vi "CodeSelet.vi"(11 "parameter name":string="ZP05") -> (3 "readData":string)   [LabVIEW 2013]
uses:
  <vilib>/addons/database/Auxilliary.llb/DB Tools Parameter Dir.ctl
  <vilib>/addons/database/Auxilliary.llb/DB Tools DataTypes.ctl
  <vilib>/addons/database/_DB Variant To Data/Database Variant To Data.xnode
  <vilib>/addons/database/NI_Database_API.lvlib
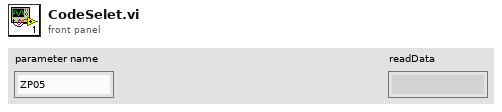
[diagram p1: front panel]
types:
  T1 = typedef "NI_Database_API.lvlib/DB Tools DataTypes.ctl" = enum16{"String", "Long (I32)", "Single (SGL)", "Double (DBL)", "Date/Time", "Binary"}
  T2 = typedef "NI_Database_API.lvlib/DB Tools Parameter Dir.ctl" = enum32{"Input", "Output", "Input/Output", "Return Value"}
  T3 = cluster{"parameter name":string, "type":T1, "direction":T2, "parameter name":string}
  T4 = cluster{"parameter name":string, "type":T1, "direction":T2, "parameter name":string}[]
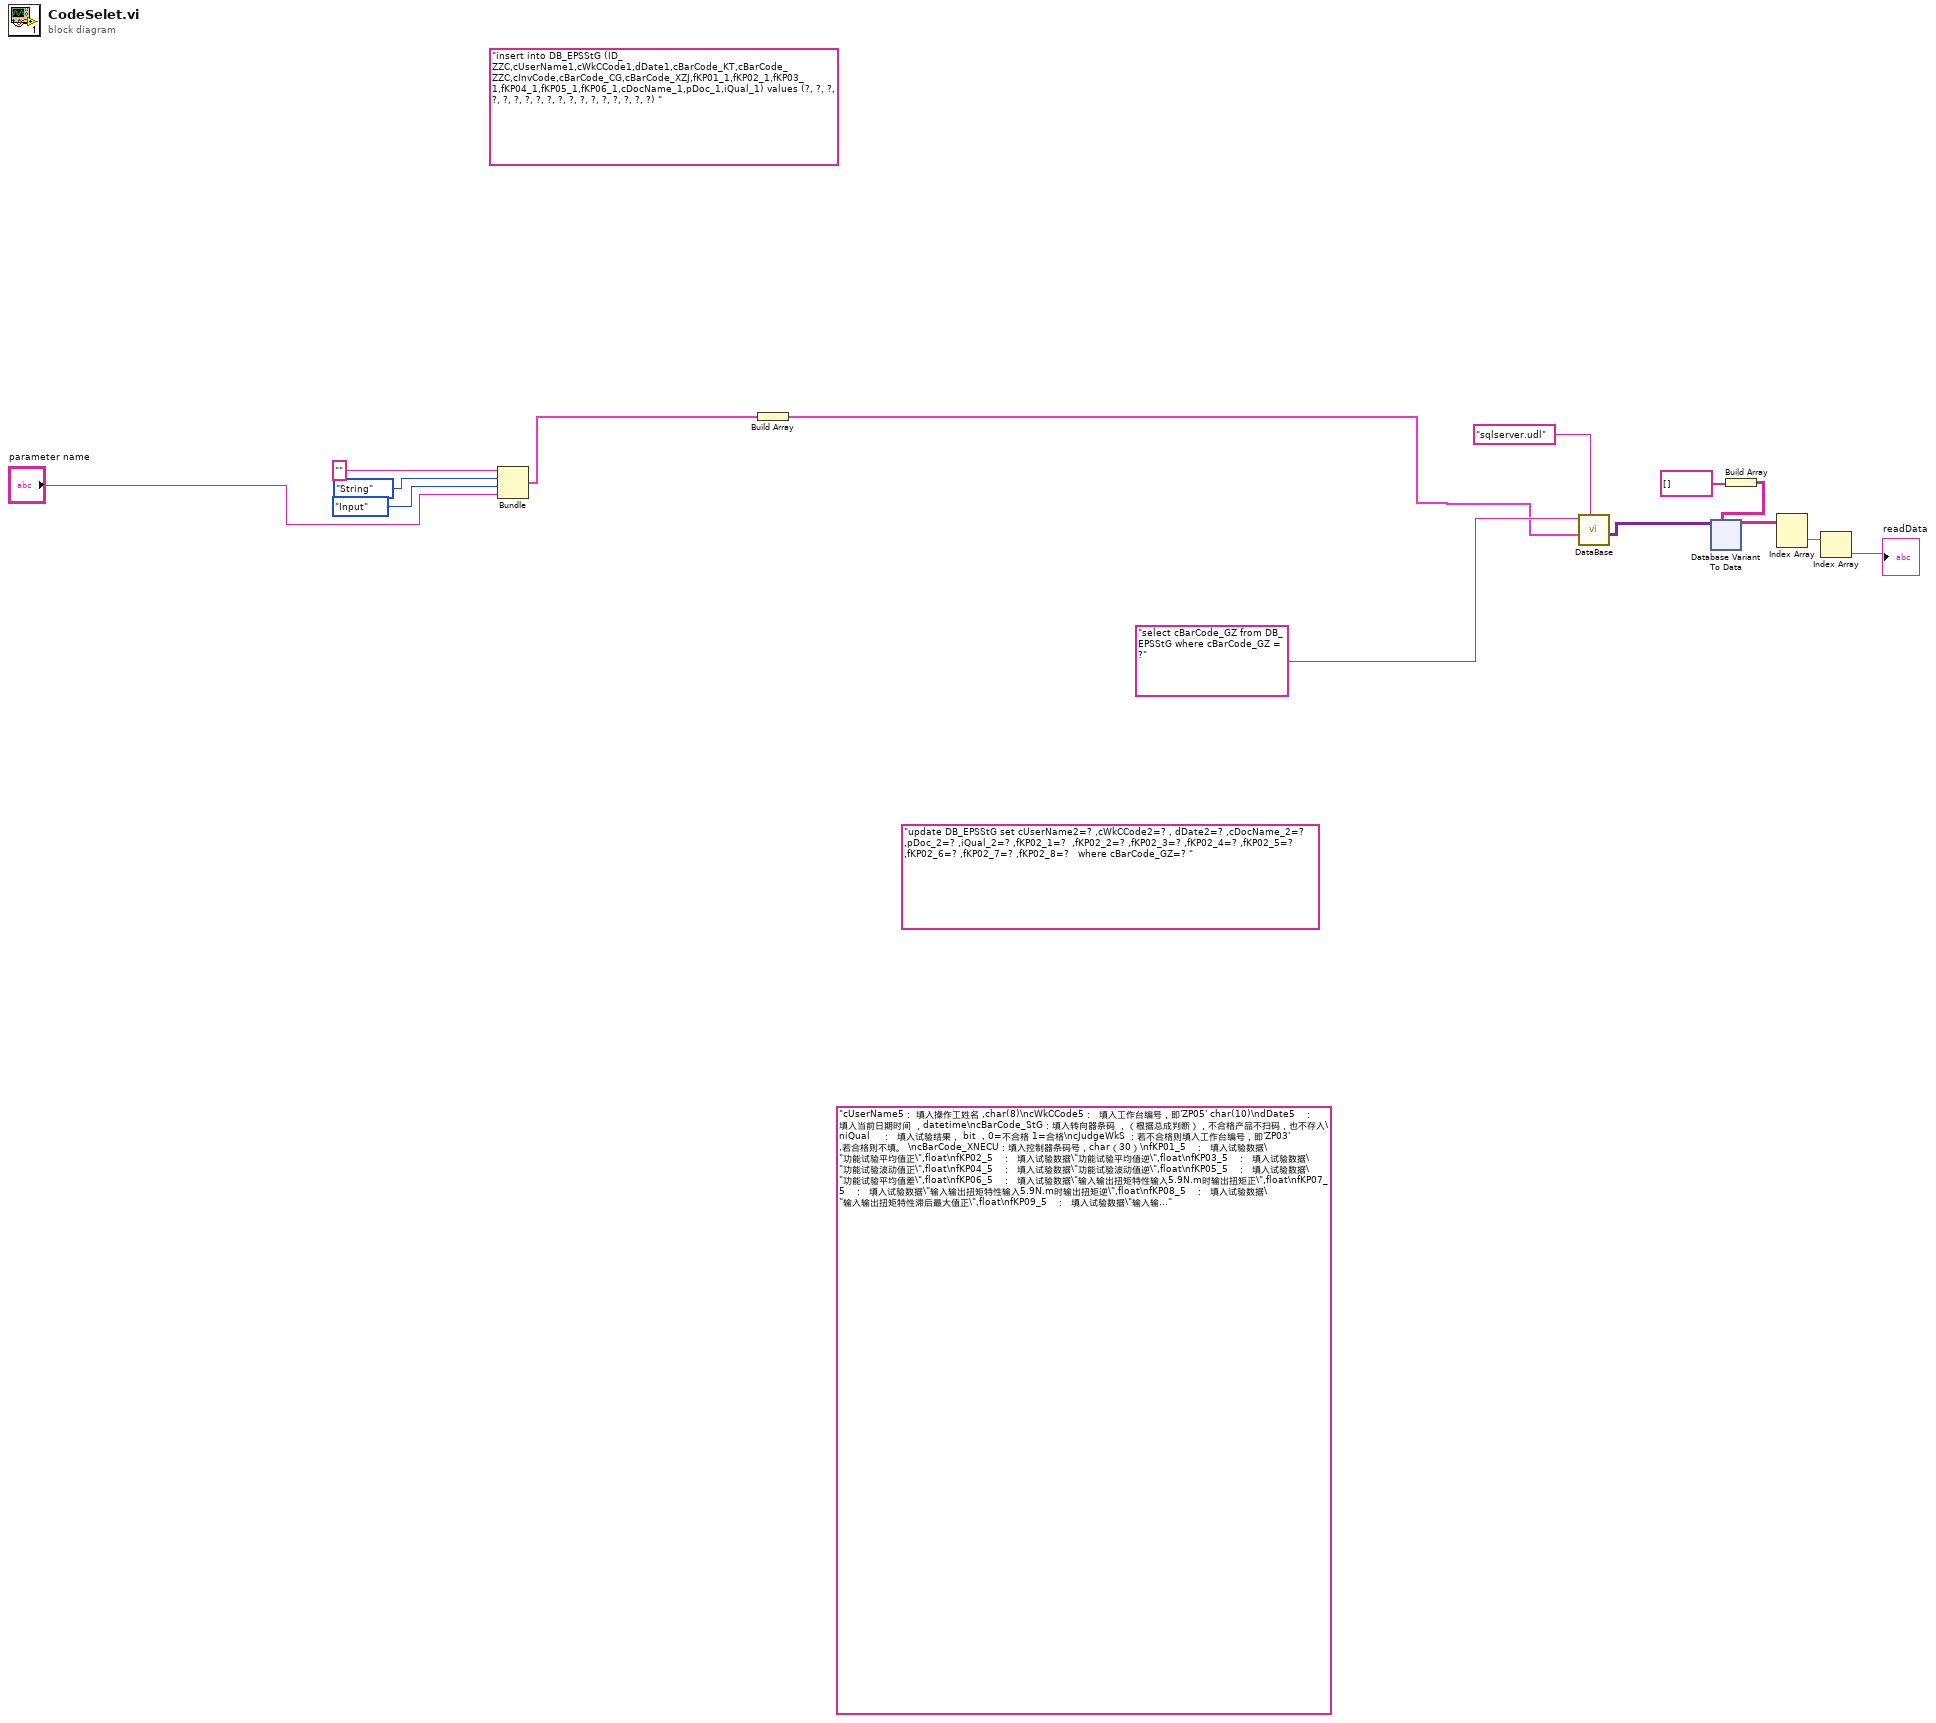
[diagram p0: block diagram]
diagram:
  (unwired) "insert into DB_EPSStG (ID_ZZC,cUserName1,cWkCCode1,dDate1,cBarCode_KT,cBarCode_ZZC,cInvCode,cBarCode_CG,cBarCode_XZJ,fKP01_1,fKP02_1,fKP03_1,fKP04_1,fKP05_1,fKP06_1,cDocName_1,pDoc_1,iQual_1) values (?, ?, ?, ?, ?, ?, ?, ?, ?, ?, ?, ?, ?, ?, ?, ?, ?, ?) " ("SQL query")
  (unwired) "update DB_EPSStG set cUserName2=? ,cWkCCode2=? , dDate2=? ,cDocName_2=? ,pDoc_2=? ,iQual_2=? ,fKP02_1=?  ,fKP02_2=? ,fKP02_3=? ,fKP02_4=? ,fKP02_5=? ,fKP02_6=? ,fKP02_7=? ,fKP02_8=?   where cBarCode_GZ=? " ("SQL query")
  (unwired) "cUserName5： 填入操作工姓名 ,char(8)\ncWkCCode5：  填入工作台编号，即'ZP05' char(10)\ndDate5   ：  填入当前日期时间 ，datetime\ncBarCode_StG：填入转向器条码 ，（根据总成判断），不合格产品不扫码，也不存入\niQual    ：  填入试验结果， bit  , 0=不合格 1=合格\ncJudgeWkS ：若不合格则填入工作台编号，即'ZP03' ,若合格则不填。 \ncBarCode_XNECU：填入控制器条码号，char（30）\nfKP01_5   ：  填入试验数据\"功能试验平均值正\",float\nfKP02_5   ：  填入试验数据\"功能试验平均值逆\",float\nfKP03_5   ：  填入试验数据\"功能试验波动值正\",float\nfKP04_5   ：  填入试验数据\"功能试验波动值逆\",float\nfKP05_5   ：  填入试验数据\"功能试验平均值差\",float\nfKP06_5   ：  填入试验数据\"输入输出扭矩特性输入5.9N.m时输出扭矩正\",float\nfKP07_5   ：  填入试验数据\"输入输出扭矩特性输入5.9N.m时输出扭矩逆\",float\nfKP08_5   ：  填入试验数据\"输入输出扭矩特性滞后最大值正\",float\nfKP09_5   ：  填入试验数据\"输入输出扭矩特性滞后最大值逆\",float\nfKP10_5   ：  填入试验数据\"输入输出扭矩特性对称度\",float\nfKP11_5   ：  填入试验数据\"扭矩传感器特性滞后最大值正\",float\nfKP12_5   ：  填入试验数据\"扭矩传感器特性滞后最大值逆\",float\nfKP13_5   ：  填入试验数据\"扭矩传感器特性对称度\",float\nfKP14_5   ：  填入试验数据\"空载平均值正\",float\nfKP15_5   ：  填入试验数据\"空载平均值逆\",float\nfKP16_5   ：  填入试验数据\"空载平均值差\",float\nfKP17_5   ：  填入试验数据\"空载波动值正\",float\nfKP18_5   ：  填入试验数据\"空载波动值逆\",float\nfKP19_5   ：  填入试验数据\"空载最大值正\",float\nfKP20_5   ：  填入试验数据\"空载最大值逆\",float\n\ncDocName_5：  填入试验报告文件名称，char（40），根据实际文件名，可与本机存储的文件名相同。\npDoc_5    ：  写入试验报告， image ,  实际的试验报告文件 \n     iQual_5   ：  填入试验结果， bit  , 0=不合格 1=合格\n" ("SQL query")
  n1 = Bundle("parameter name"="", "type"=DB_Tools_DataTypes."String", "direction"=DB_Tools_Parameter_Dir."Input", "parameter name"="parameter name") -> (w10:T3)  [unwired: 1 in]
  n2 = Build Array(w10) -> (w2:T4)
  n3 = call "DataBase.vi"("udl名称"="sqlserver.udl", "parameters"=w2, "SQL query"="select cBarCode_GZ from DB_EPSStG where cBarCode_GZ = ?") -> ("recordset data"=w4:variant[][])  [unwired: 8 in]
  n4 = Build Array(string[] [] ("添加的数组")) -> (w7:string[][])
  n5 = xnode "Database Variant To Data"("database variant"=w4, "type"=w7) -> ("data"=w5:string[][])  [unwired: 1 in, 1 out]
  n6 = Index Array(array=w5) -> (element=w6:string[])  [unwired: 2 in]
  n7 = Index Array(array=w6) -> (element=→"readData":string)  [unwired: 1 in]
